vi "Process Protection Signals.vi"(0 "Frame Settings In":T2 {"Protection Configurations"."CRC Channels"."Data Type" items=["Signed", "Unsigned", "IEEE Float"]}, 1 "Incoming Values In":T1, 2 "Values Received":dbl[](array[numeric]), 3 "error in (no error)":errorcluster) -> (7 "Frame Settings Out":T2 {"Protection Configurations"."CRC Channels"."Data Type" items=["Signed", "Unsigned", "IEEE Float"]}, 8 "Incoming Values Out":T1, 10 "error out":errorcluster)   [LabVIEW 2019, in "Protection and Counter Addon Engine.lvlib"]
uses:
  Protection and Counter Addon Engine.lvlib
  SubModules/Frame-Protection-Support/Source/Engine/Types/RT Frame Settings.ctl
  SubModules/Frame-Protection-Support/Source/Shared/Types/Exported Frame Type.ctl
  SubModules/Frame-Protection-Support/Source/Engine/Types/RT Protection Configuration.ctl
  SubModules/Frame-Protection-Support/Source/Shared/Types/Protection Type.ctl
  SubModules/Frame-Protection-Support/Source/Shared/Types/XNET Signal Configuration.ctl
  SubModules/Frame-Protection-Support/Source/Shared/Types/Exported Counter Settings.ctl
  SubModules/Frame-Protection-Support/Source/Shared/Types/Exported Event Trigger Type.ctl
  Types/Incoming Values.ctl
  SubModules/Frame-Protection-Support/Source/Engine/SubVIs/Get Protection Signals.vi
  <vilib>/xnet/xnet.llb/XNET Convert.vi
  <vilib>/xnet/xnet.llb/XNET Convert (Signal to Frame Raw).vi
  SubModules/Frame-Protection-Support/Source/Engine/Protection and Counter Support Engine.lvlib
  SubModules/Frame-Protection-Support/Source/Shared/Protection and Counter Support Shared.lvlib
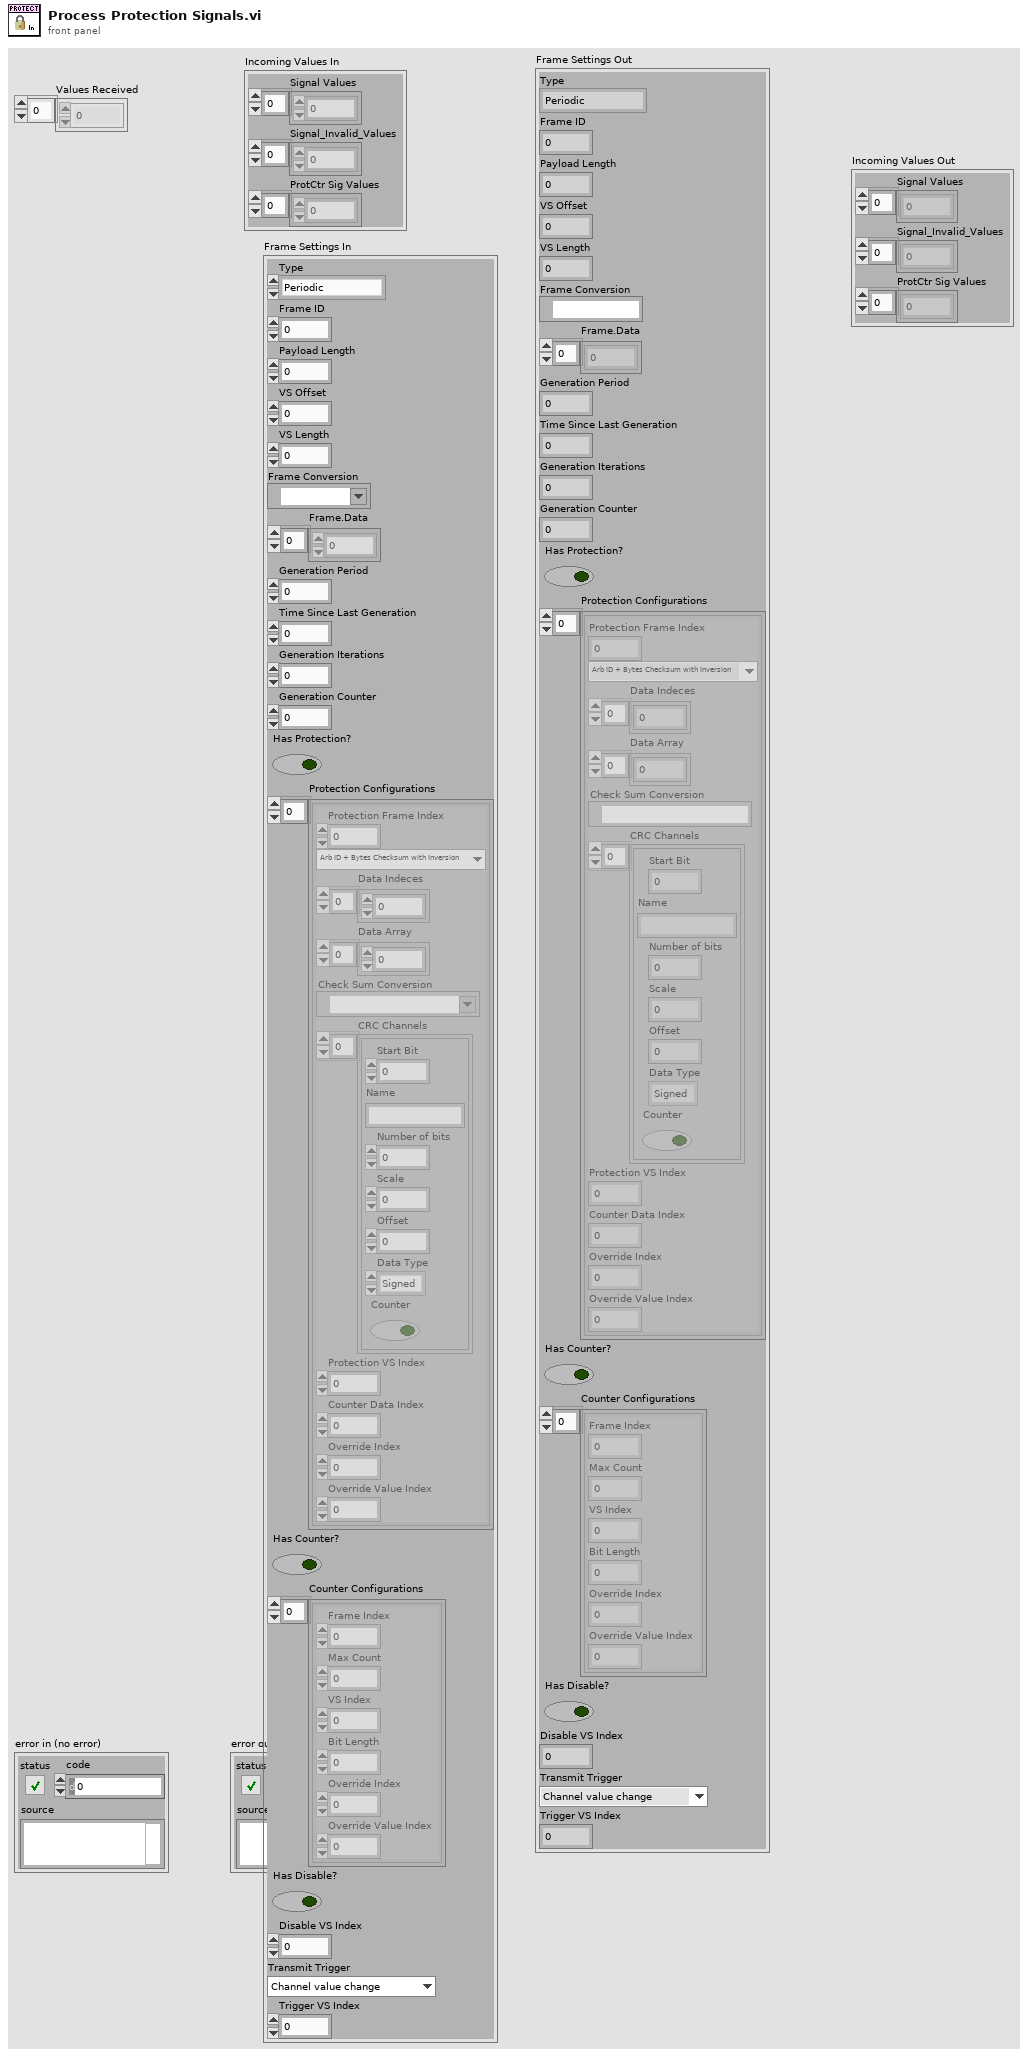
[diagram p1: front panel]
types:
  T1 = typedef "Incoming Values.ctl" = cluster{"Signal Values":dbl[], "Signal_Invalid_Values":dbl[], "ProtCtr Sig Values":dbl[]}
  T2 = typedef "Protection and Counter Support Engine.lvlib/RT Frame Settings.ctl" = cluster{"Type":T3, "Frame ID":u32, "Payload Length":u32, "VS Offset":i32, "VS Length":i32, "Frame Conversion":refnum<k21>, "Frame.Data":dbl[], "Generation Period":u32, "Time Since Last Generation":u32, "Generation Iterations":u32, "Generation Counter":u32, "Has Protection?":bool, "Protection Configurations":T4[], "Has Counter?":bool, "Counter Configurations":T7[], "Has Disable?":bool, "Disable VS Index":i32, "Transmit Trigger":T8, "Trigger VS Index":i32}
  T3 = typedef "Protection and Counter Support Shared.lvlib/Exported Frame Type.ctl" = enum16{"Periodic", "Event", "Periodic/Event"}
  T4 = typedef "Protection and Counter Support Engine.lvlib/RT Protection Configuration.ctl" = cluster{"Protection Frame Index":i32, "Protection Type":T5, "Data Indeces":i32[], "Data Array":dbl[], "Check Sum Conversion":refnum<k21>, "CRC Channels":T6[], "Protection VS Index":i32, "Counter Data Index":i32, "Override Index":i32, "Override Value Index":i32}
  T5 = typedef "Protection and Counter Support Shared.lvlib/Protection Type.ctl" = enum16{"Arb ID + Bytes Checksum with Inversion", "Arb ID + Bytes CRC with Inversion", "Reversed Raw Signal Checksum with Inversion", "Concatenated Two's Compliment"}
  T6 = typedef "Protection and Counter Support Shared.lvlib/XNET Signal Configuration.ctl" = cluster{"Start Bit":i32, "Name":string, "Number of bits":i32, "Scale":dbl, "Offset":dbl, "Data Type":u32, "Counter":bool}
  T7 = typedef "Protection and Counter Support Shared.lvlib/Exported Counter Settings.ctl" = cluster{"Frame Index":i32, "Max Count":dbl, "VS Index":i32, "Bit Length":i64, "Override Index":i32, "Override Value Index":i32}
  T8 = typedef "Protection and Counter Support Shared.lvlib/Exported Event Trigger Type.ctl" = enum16{"Channel value change", "Trigger channel (not zero)", "Channel value change or trigger channel (not zero)", "Trigger channel (any value change)", "Channel value change or trigger channel (any value change)"}
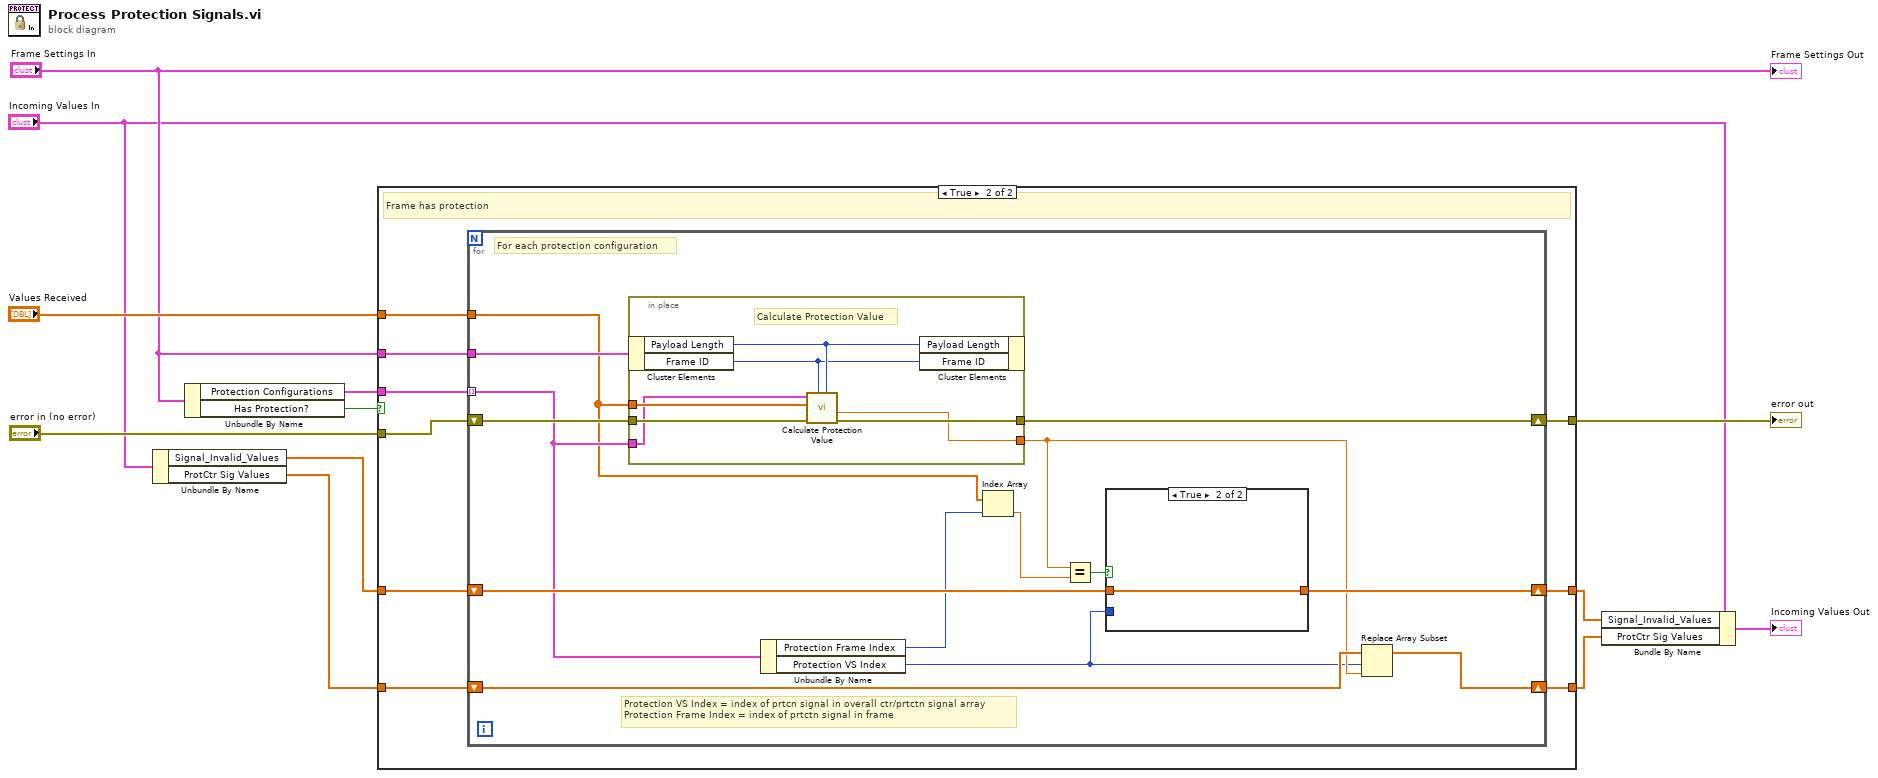
[diagram p0: block diagram]
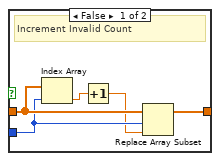
[diagram p3: hidden frame]
diagram:
  n1 = Unbundle By Name("Incoming Values In") -> ("Signal_Invalid_Values"=w4:dbl[], "ProtCtr Sig Values"=w3:dbl[])
  n2 = Unbundle By Name("Frame Settings In") -> ("Protection Configurations"=w7:T4[], "Has Protection?"=w11:bool)
  n3 = case shown="True" w11 {
    tunnel: "error in (no error)" -> [w15 w18]
    tunnel: [w15 w19] -> w10
    tunnel: "Frame Settings In" -> [_ w20]
    tunnel: w4 -> [w13 w24]
    tunnel: [w13 w23] -> w2
    tunnel: w3 -> [w14 w22]
    tunnel: [w14 w21] -> w1
    tunnel: "Values Received" -> [_ w17]
    tunnel: w7 -> [_ w16]
    frame False {
      # "Frame does not have protection"
    }
    frame True {
      # "Frame has protection"
      n4 = for {
        tunnel: w20 -> [w34]
        tunnel: w17 -> [w28]
        shift-right: [w33] -> w19
        shift-left: w18 -> [w32]
        tunnel: w16 -> [w29] mode=indexing
        shift-right: [w37] -> w23
        shift-left: w24 -> [w38]
        shift-right: [w35] -> w21
        shift-left: w22 -> [w36]
        # "Protection VS Index = index of prtcn signal in overall ctr/prtctn signal array\nProtection Frame Index = index of prtctn signal in frame"
        # "For each protection configuration"
        n5 = in-place {
          in-place-border: w32 -> [w51]
          in-place-border: [w48] -> w33
          in-place-border: w28 -> [w47]
          in-place-border: [w46] -> w31
          in-place-border: w29 -> [w45]
          # "Calculate Protection Value"
          n6 = in-place-cluster #1(w34) -> ("Payload Length"=w50:u32, "Frame ID"=w49:u32)
          n7 = call "Calculate Protection Value.vi"("Payload Length"=w50, "Frame ID"=w49, "error in (no error)"=w51, "Frame.Data in"=w47, "Protection Configuration in"=w45) -> ("error out"=w48:errorcluster, "Protection Value"=w46:dbl)  [unwired: 3 in, 2 out]
          n8 = in-place-cluster #1("Payload Length"=w50, "Frame ID"=w49) -> ()  [unwired: 1 out]
        }
        n9 = Unbundle By Name(w29) -> ("Protection Frame Index"=w25:i32, "Protection VS Index"=w27:i32)
        n10 = Index Array(array=w28, index=w25) -> (element=w26:dbl)
        n11 = Equal?(x=w31, y=w26) -> (x = y?=w30:bool)
        n12 = case shown="True" w30 {
          tunnel: w38 -> [w42 w44]
          tunnel: [w43 w44] -> w37
          tunnel: w27 -> [w41 _]
          frame False {
            # "Increment Invalid Count"
            n13 = Index Array(array=w42, index=w41) -> (element=w40:dbl)
            n14 = Increment(x=w40) -> (x+1=w39:dbl)
            n15 = Replace Array Subset(array=w42, new element=w39, index=w41) -> (w43:dbl[])
          }
          frame True {
          }
        }
        n16 = Replace Array Subset(array=w36, new element=w31, index=w27) -> (w35:dbl[])
      }
    }
  }
  "error out" <- w10
  n17 = Bundle By Name(cluster="Incoming Values In", "Signal_Invalid_Values"=w2, "ProtCtr Sig Values"=w1) -> (→"Incoming Values Out":T1)
  "Frame Settings Out" <- "Frame Settings In"
